vi "Read Double.vi"(7 "Channel Array in":refnum<class "CIFChannels.lvclass">[](array[class]), 8 "error in (no error)":errorcluster, 10 "Channel Index":i32) -> (0 "error out":errorcluster, 1 "timed out?":bool, 2 "Data":dbl, 5 "Channel Array out":refnum<class "CIFChannels.lvclass">[](array[class]))   [LabVIEW 2021, in "CIFChannelMng.lvclass"]
uses:
  CIFChannelMng.lvclass
  <vilib>/CIF Foundation/CIF Channels Core/CIFChannels/CIFChannels.lvclass
  CIFChannelMng.lvclass/CIFChannelMng.ctl
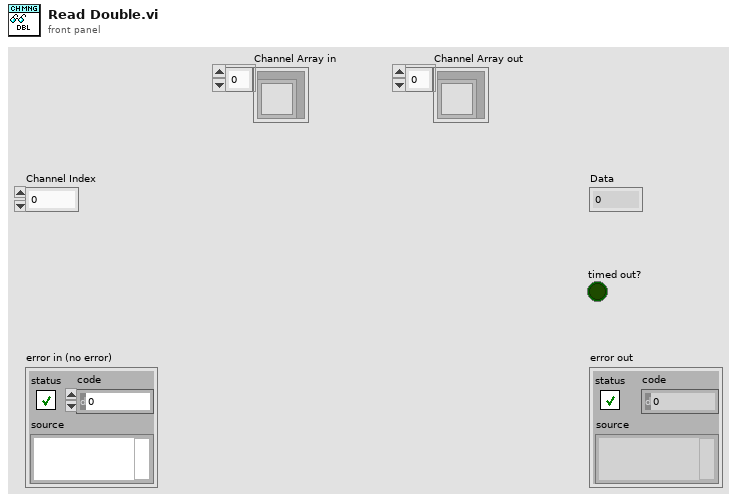
[diagram p1: front panel]
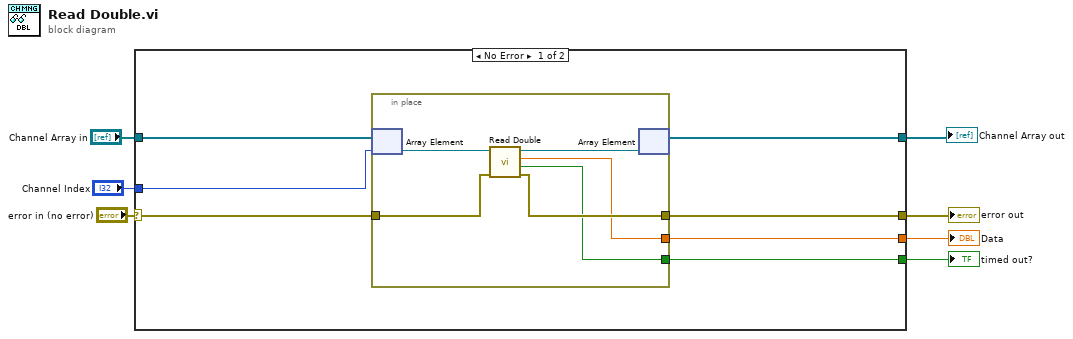
[diagram p0: block diagram]
diagram:
  n1 = case shown="No Error" "error in (no error)" {
    selector: "error in (no error)" -> [w14 w22]
    tunnel: [w13 w22] -> w6
    tunnel: [w12 _] -> w5
    tunnel: [w11 _] -> w4
    tunnel: "Channel Index" -> [w10 _]
    tunnel: "Channel Array in" -> [w9 w21]
    tunnel: [w8 w21] -> w1
    frame No Error {
      n2 = in-place {
        in-place-border: w14 -> [w20]
        in-place-border: [w19] -> w13
        in-place-border: [w18] -> w11
        in-place-border: [w17] -> w12
        n3 = in-place-array #1(w9, w10) -> (w16:refnum<class "CIFChannels.lvclass">)
        n4 = call-dynamic "Read Double.vi"("error in (no error)"=w20, "CIFChannels in"=w16) -> ("error out"=w19:errorcluster, "timed out?"=w18:bool, "Data"=w17:dbl, "CIFChannels out"=w15:refnum<class "CIFChannels.lvclass">)  [unwired: 6 in]
        n5 = in-place-array #1(w15) -> (w8:refnum<class "CIFChannels.lvclass">[])  [unwired: 1 out]
      }
    }
    frame Error {
    }
  }
  "error out" <- w6
  "Data" <- w5
  "timed out?" <- w4
  "Channel Array out" <- w1
